vi "testPixelflySequence.vi"() -> ()   [LabVIEW 2009, in "run.lvlib"]
uses:
  testing/run.lvlib
panel:
  out "Number taken":i32
  out "Image":T1(plugin-control)
  in  "number of images":i32=1
  in  "stop":bool
  out "Board Parameters":T2 {"Vertical bin" items=["1", "2"]; "Horizontal bin" items=["1", "2"]}
  in  "gain":i32(ring) items=["Low (X1)", "High (X2)"]
  in  "exp time":i32(slide)=36 min=1 max=10000 scale=0.0..500.0
  in  "V bin":i32(ring) items=["1", "2"]
  in  "H bin":i32(ring) items=["1", "2"]
  in  "trigger":bool
  in  "Exposure mode":u16(ring)=2 items=["Asynch shutter", "Double shot", "Video mode", "Auto exposure"]
  out "ccdtemp":i32(slide) scale=0.0..100.0
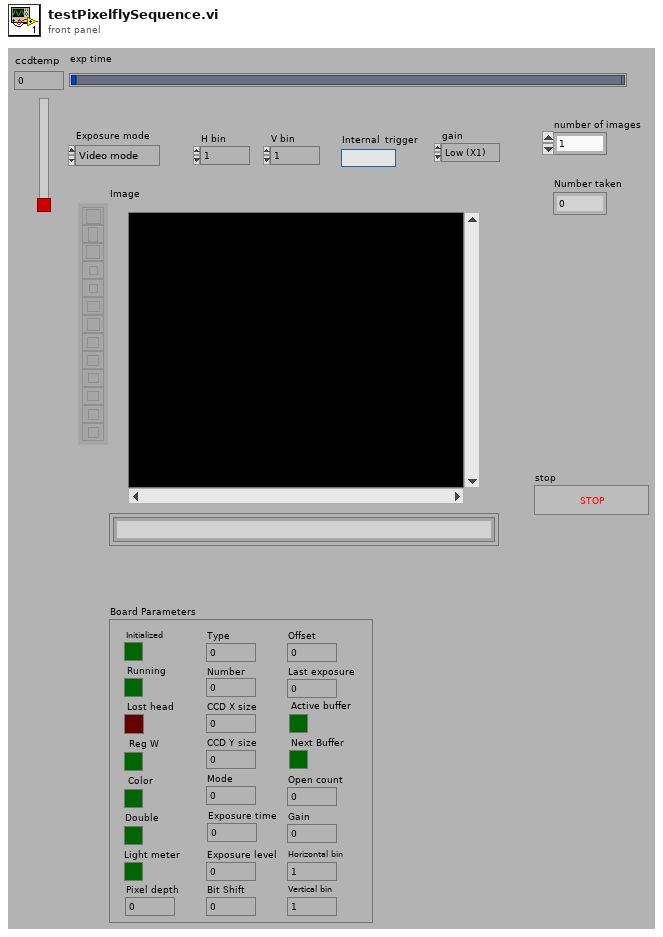
[diagram p1: front panel]
types:
  T1 = typedef "IMAQ Image.ctl" = refnum<image>
  T2 = cluster{"Type":u32, "Number":u32, "Initialized":bool, "Running":bool, "Lost head":bool, "CCD X size":u32, "CCD Y size":u32, "Mode":u32, "Exposure time":u32, "Exposure level":u32, "Horizontal bin":u32, "Vertical bin":u32, "Reg W":bool, "Gain":u32, "Pixel depth":i32, "Bit Shift":u32, "Offset":u32, "Last exposure":u32, "Double ":bool, "Light meter":bool, "Color":bool, "Open count":u32, "Active buffer":bool, "Next Buffer":bool}
  T3 = typedef "Image Type" = u32
  T4 = cluster{"ccdxsize":i32, "ccdy":i32, "pictx":i32, "picty":i32, "bitspixel":i32}
  T5 = cluster{"Write":bool, "Write done":bool, "Queued":bool, "Cancelled":bool, "Select":bool, "Select done":bool, "Burst":bool, "Size":bool, "Event":bool, "Timeout":bool, "Open":i32, "Map":i32, "Exposure":i32[], "Offset":i32[], "Size":i32[], "Transfer":i32[], "Total Size":i32}
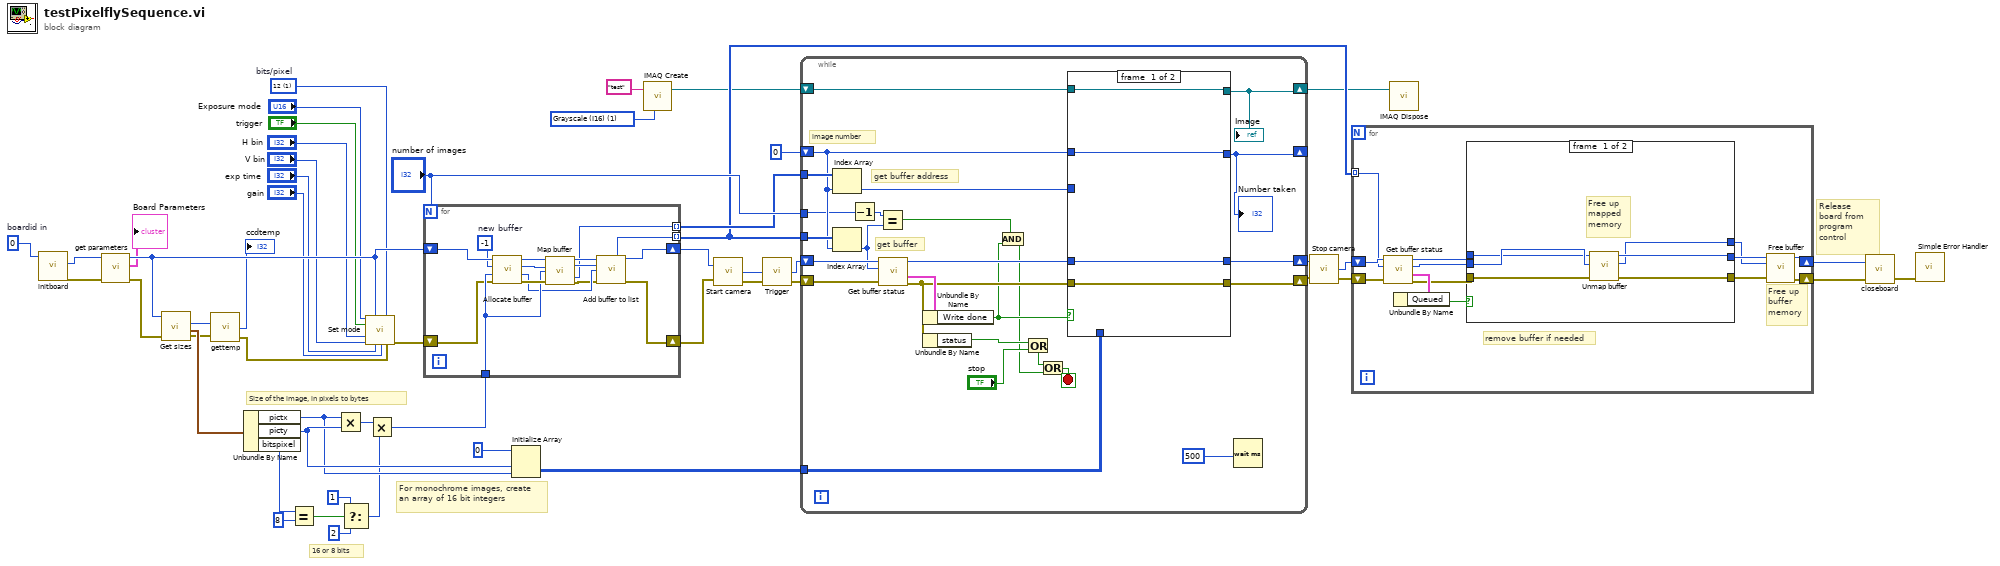
[diagram p0: block diagram]
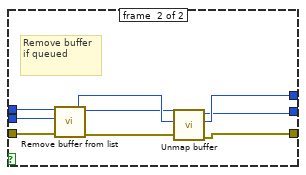
[diagram p2: hidden frame]
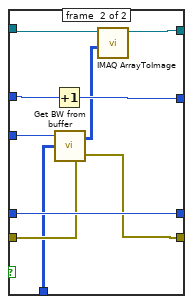
[diagram p3: hidden frame]
diagram:
  w4 = T3 1 items=["Grayscale (U8)", "Grayscale (I16)", "Grayscale (SGL)", "Complex (CSG)", "RGB (U32)", "HSL (U32)", "RGB (U64)", "Grayscale (U16)"] ("Image Type")
  w25 = 1 items=["8", "12"]  # bits/pixel
  w35 = 0  # boardid in
  # "Release board from program control"
  # "16 or 8 bits"
  # "For monochrome images, create an array of 16 bit integers"
  # "Size of the image, in pixels to bytes"
  n1 = call <instrlib>:"initboard.vi"("boardid in"=w35) -> ("boardid"=w51:i32, "error out"=w24:errorcluster)  [unwired: 3 in, 1 out]
  n2 = call <instrlib>:"get parameters.vi"("error in (no error)"=w24, "Handle in"=w51) -> ("error out"=w39:errorcluster, "Board Parameters"=→"Board Parameters":T2, "Error out"=w36:i32)  [unwired: 2 in, 1 out]
  n3 = call <instrlib>:"Get sizes.vi"("Handle in"=w36, "error in (no error)"=w39) -> ("Handle out"=w37:i32, "Picture parameters"=w47:T4, "error out"=w38:errorcluster)  [unwired: 1 in, 1 out]
  n4 = call <instrlib>:"gettemp.vi"("Handle in"=w37, "error in (no error)"=w38) -> ("ccdtemp"=→"ccdtemp":i32, "error out"=w52:errorcluster)  [unwired: 1 out]
  n5 = Unbundle By Name(w47) -> ("pictx"=w44:i32, "picty"=w45:i32, "bitspixel"=w46:i32)
  n6 = Equal?(x=w46, y=8) -> (x = y?=w43:bool)
  n7 = Multiply(x=w44, y=w45) -> (x*y=w49:i32)
  n8 = Select(t=1, s=w43, f=2) -> (s? t:f=w40:i32)
  n9 = call <instrlib>:"Set mode.vi"("Exposure mode"="Exposure mode", "Handle in"=w36, "bits/pixel"=w25, "trigger"="trigger", "H bin"="H bin", "V bin"="V bin", "exp time"="exp time", "gain"="gain", "error in (no error)"=w52) -> ("error out"=w33:errorcluster)  [unwired: 6 in]
  n10 = Multiply(x=w49, y=w40) -> (x*y=w34:i32)
  n11 = for {
    N: "number of images" -> [_]
    tunnel: w34 -> [w64]
    shift-right: [w55] -> w22
    shift-left: w36 -> [w65]
    shift-right: [w56] -> w21
    shift-left: w33 -> [w63]
    tunnel: [w54] -> w8 mode=indexing
    tunnel: [w53] -> w16 mode=indexing
    w62 = -1  # new buffer
    n12 = call <instrlib>:"Allocate buffer.vi"("error in (no error)"=w63, "Size request"=w64, "Buffer request"=w62, "Handle in"=w65) -> ("error out"=w66:errorcluster, "Size"=w58:i32, "Buffer number"=w61:i32, "Handle out"=w67:i32)
    n13 = call <instrlib>:"Map buffer.vi"("Handle in"=w67, "Buffer in"=w61, "size"=w64, "error in (no error)"=w66) -> ("Handle out"=w60:i32, "Buffer number"=w59:i32, "Buffer address"=w53:i32, "error out"=w57:errorcluster)  [unwired: 8 in]
    n14 = call <instrlib>:"Add buffer to list.vi"("Handle in"=w60, "Buffer in"=w59, "size"=w58, "error in (no error)"=w57) -> ("Buffer number"=w54:i32, "Handle out"=w55:i32, "error out"=w56:errorcluster)  [unwired: 9 in]
  }
  n15 = Initialize Array(u16 0 ("16 bit integers"), w45, w44) -> (w6:u16[][])
  n16 = call "IMAQ Create"("Image Name"="test", "Image Type"=w4) -> ("New Image"=w5:T1)  [unwired: 3 in, 1 out]
  n17 = call <instrlib>:"Start camera.vi"("Handle in"=w22, "error in (no error)"=w21) -> ("Handle out"=w20:i32, "error out"=w19:errorcluster)  [unwired: 1 out]
  n18 = call <instrlib>:"Trigger.vi"("Handle in"=w20, "error in (no error)"=w19) -> ("Handle out"=w18:i32, "error out"=w1:errorcluster)  [unwired: 1 out]
  n19 = while {
    shift-right: [w85] -> w14
    shift-left: w18 -> [w82]
    shift-right: [w84] -> w13
    shift-left: w1 -> [w91]
    tunnel: w8 -> [w81]
    tunnel: "number of images" -> [w73]
    tunnel: w16 -> [w79]
    tunnel: w6 -> [w83]
    shift-right: [w69] -> _
    shift-left: 0 -> [w78]
    shift-right: [w75] -> w2
    shift-left: w5 -> [w76]
    stop <- w89 stop-if-true
    # "get buffer address"
    # "image number"
    # "get buffer"
    n20 = Index Array(array=w79, index=w78) -> (element=w77:i32)
    n21 = Index Array(array=w81, index=w78) -> (element=w80:i32)
    n22 = Decrement(x=w73) -> (x-1=w74:i32)
    n23 = Equal?(x=w74, y=w80) -> (x = y?=w72:bool)
    n24 = call <instrlib>:"Get buffer status.vi"("error in (no error)"=w91, "Buffer request"=w80, "Handle in"=w82) -> ("error out"=w86:errorcluster, "Buffer status"=w93:T5, "Handle out"=w87:i32)  [unwired: 1 in, 1 out]
    n25 = Unbundle By Name(w93) -> ("Write done"=w71:bool)
    n26 = Unbundle By Name(w86) -> ("status"=w88:bool)
    n27 = And(x=w72, y=w71) -> (x .and. y?=w70:bool)
    n28 = Or(x=w88, y="stop") -> (x .or. y?=w90:bool)
    n29 = Or(x=w90, y=w70) -> (x .or. y?=w89:bool)
    n30 = case shown="True" w71 {
      tunnel: w87 -> [w97 w107]
      tunnel: w86 -> [w96 w106]
      tunnel: [w97 w107] -> w85
      tunnel: [w96 w105] -> w84
      tunnel: w77 -> [_ w104]
      tunnel: w83 -> [_ w103]
      tunnel: w78 -> [w95 w102]
      tunnel: [w95 w101] -> w69
      tunnel: w76 -> [w94 w100]
      tunnel: [w94 w98] -> w75
      frame #0 {
      }
      frame #1 {
        n31 = Increment(x=w102) -> (x+1=w101:i32)
        n32 = call <instrlib>:"Get BW from buffer.vi"("error in (no error)"=w106, "Array input"=w103, "Buffer address"=w104) -> ("error out"=w105:errorcluster, "Image data"=w99:u16[][])
        n33 = call "IMAQ ArrayToImage"("Image Pixels (I16)"=w99, "Image"=w100) -> ("Image Out"=w98:T1)  [unwired: 8 in, 1 out]
      }
    }
    "Image" <- w75
    "Number taken" <- w69
    n34 = Wait (ms)(milliseconds to wait=500) -> ()  [unwired: 1 out]
  }
  n35 = call <instrlib>:"Stop camera.vi"("Handle in"=w14, "error in (no error)"=w13) -> ("Handle out"=w10:i32, "error out"=w9:errorcluster)  [unwired: 1 out]
  n36 = for {
    shift-right: [w115] -> w11
    shift-left: w10 -> [w110]
    shift-right: [w120] -> w12
    shift-left: w9 -> [w109]
    tunnel: w8 -> [w108] mode=indexing
    # "remove buffer if needed"
    # "Free up buffer memory"
    n37 = call <instrlib>:"Get buffer status.vi"("error in (no error)"=w109, "Buffer request"=w108, "Handle in"=w110) -> ("error out"=w118:errorcluster, "Buffer status"=w119:T5, "Buffer number"=w117:i32, "Handle out"=w116:i32)  [unwired: 1 in]
    n38 = Unbundle By Name(w119) -> ("Queued"=w114:bool)
    n39 = case shown="True" w114 {
      tunnel: w118 -> [w122 w135]
      tunnel: [w125 w129] -> w111
      tunnel: w117 -> [w126 w134]
      tunnel: w116 -> [w121 w133]
      tunnel: [w124 w130] -> w113
      tunnel: [w123 w131] -> w112
      frame #0 {
        # "Free up mapped memory"
        n40 = call <instrlib>:"Unmap buffer.vi"("error in (no error)"=w122, "Buffer in"=w126, "Handle in"=w121) -> ("error out"=w125:errorcluster, "Buffer number"=w123:i32, "Handle out"=w124:i32)  [unwired: 2 in]
      }
      frame #1 {
        # "Remove buffer if queued"
        n41 = call <instrlib>:"Remove buffer from list.vi"("error in (no error)"=w135, "Buffer in"=w134, "Handle in"=w133) -> ("error out"=w128:errorcluster, "Buffer number"=w132:i32, "Handle out"=w127:i32)  [unwired: 2 in]
        n42 = call <instrlib>:"Unmap buffer.vi"("error in (no error)"=w128, "Buffer in"=w132, "Handle in"=w127) -> ("error out"=w129:errorcluster, "Buffer number"=w131:i32, "Handle out"=w130:i32)  [unwired: 2 in]
      }
    }
    n43 = call <instrlib>:"Free buffer.vi"("error in (no error)"=w111, "Buffer in"=w112, "Handle in"=w113) -> ("error out"=w120:errorcluster, "Handle out"=w115:i32)  [unwired: 2 in, 1 out]
  }
  n44 = call "IMAQ Dispose"("Image"=w2) -> ()  [unwired: 5 in, 1 out]
  n45 = call <instrlib>:"closeboard.vi"("Handle in"=w11, "error in (no error)"=w12) -> ("error out"=w7:errorcluster)  [unwired: 2 out]
  n46 = call <vilib>:"Simple Error Handler.vi"("error in (no error)"=w7) -> ()  [unwired: 4 in, 5 out]
